vi "setUp.vi"(8 "error in (no error)":errorcluster, 11 "reference in":refnum<class "FPGA Addon DMA Channels Interleaved System Tests.lvclass">=refnum) -> (0 "error out":errorcluster, 3 "reference out":refnum<class "FPGA Addon DMA Channels Interleaved System Tests.lvclass">)   [LabVIEW 2019, in "FPGA Addon DMA Channels Interleaved System Tests.lvclass"]
doc: "setUp runs prior to the test method during test execution. Use this method to initialize any object data required by your tests."
uses:
  FPGA Addon DMA Channels Interleaved System Tests.lvclass
  FPGA Addon Test Class/FPGA Addon Test Class.lvclass
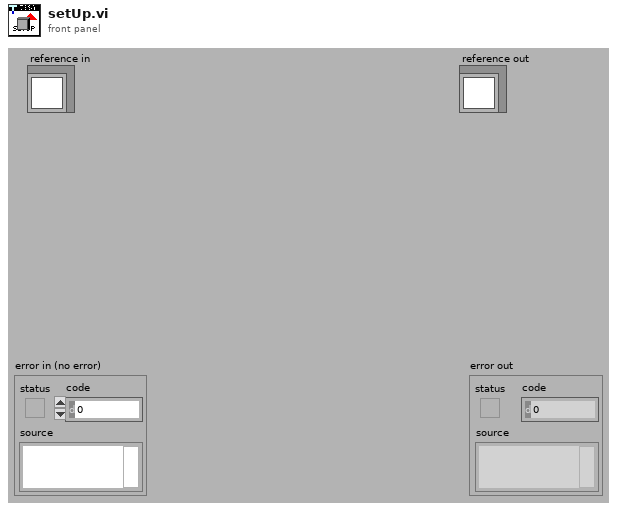
[diagram p1: front panel]
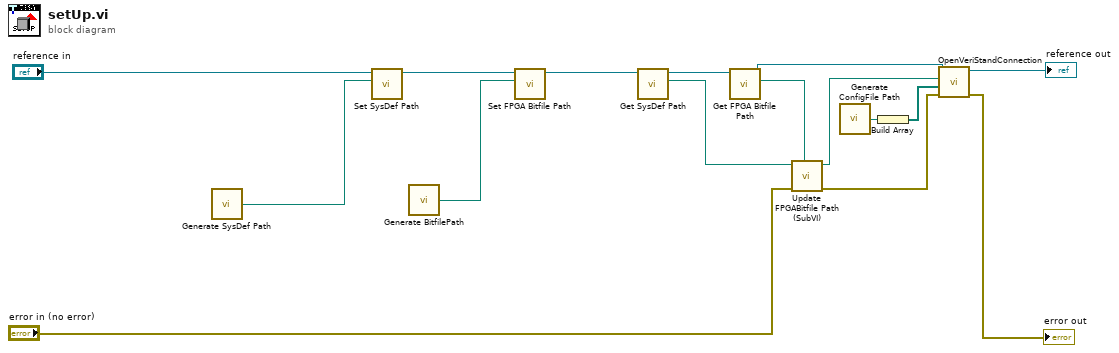
[diagram p0: block diagram]
diagram:
  n1 = call "Generate SysDef Path.vi"() -> ("SysDef path"=w10:path)
  n2 = call "Set SysDef Path.vi"("SysDef Path"=w10, "Scalar Channels Testing in"="reference in") -> ("Scalar Channels Testing out"=w16:refnum<class "FPGA Addon Test Class.lvclass">)  [unwired: 9 in]
  n3 = call "Generate BitfilePath.vi"() -> ("Bitfile path"=w9:path)
  n4 = call "Set FPGA Bitfile Path.vi"("FPGA Bitfile Path"=w9, "Scalar Channels Testing in"=w16) -> ("Scalar Channels Testing out"=w15:refnum<class "FPGA Addon Test Class.lvclass">)  [unwired: 9 in]
  n5 = call "Get SysDef Path.vi"("Scalar Channels Testing in"=w15) -> ("SysDef Path"=w12:path, "Scalar Channels Testing out"=w14:refnum<class "FPGA Addon Test Class.lvclass">)  [unwired: 9 in]
  n6 = call "Get FPGA Bitfile Path.vi"("Scalar Channels Testing in"=w14) -> ("FPGA Bitfile Path"=w13:path, "Scalar Channels Testing out"=w7:refnum<class "FPGA Addon Test Class.lvclass">)  [unwired: 9 in]
  n7 = call "Update FPGABitfile Path (SubVI).vi"("Bitfile Path"=w13, "error in (no error)"="error in (no error)", "System Definition path in"=w12) -> ("error out"=w6:errorcluster, "System Definition path out"=w4:path)  [unwired: 7 in]
  n8 = call "Generate ConfigFile Path.vi"() -> ("ConfigFile path"=w2:path)
  n9 = Build Array(w2) -> (w1:path[])
  n10 = call-dynamic "OpenVeriStandConnection.vi"("error in (no error)"=w6, "overrides files"=w1, "System Definition File"=w4, "VeriStand Test Case in"=w7) -> ("error out"=→"error out":errorcluster, "VeriStand Test Case out"=→"reference out":refnum<class "FPGA Addon DMA Channels Interleaved System Tests.lvclass">)  [unwired: 5 in, 1 out]
